vi "get_freqvals.vi"(1 "Fsample":dbl, 2 "NFFT":i32) -> (0 "FreqVals":dbl[](array[numeric]))   [LabVIEW 2019]
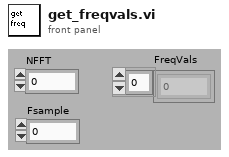
[diagram p1: front panel]
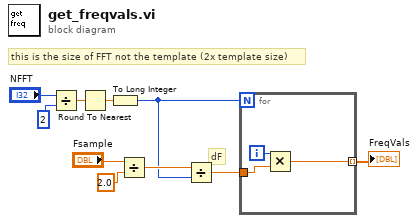
[diagram p0: block diagram]
diagram:
  # "dF"
  # "this is the size of FFT not the template (2x template size)"
  n1 = Divide(x="NFFT", y=2) -> (x/y=w7:dbl)
  n2 = Round To Nearest(number=w7) -> (nearest integer value=w8:dbl)
  n3 = To Long Integer(number=w8) -> (32bit integer=w1:i32)
  n4 = Divide(x="Fsample", y=2.0) -> (x/y=w4:dbl)
  n5 = Divide(x=w4, y=w1) -> (x/y=w3:dbl)
  n6 = for {
    N: w1 -> [_]
    tunnel: w3 -> [w12]
    tunnel: [w11] -> w2 mode=indexing
    i -> [w13]
    n7 = Multiply(x=w13, y=w12) -> (x*y=w11:dbl)
  }
  "FreqVals" <- w2
